vi "niFpgaNotchTemplate.vi"(0 "input data":fxp<+/-,16,16>) -> (4 "output data":fxp<+/-,20,20>)   [LabVIEW 2017]
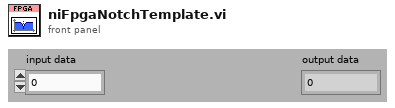
[diagram p1: front panel]
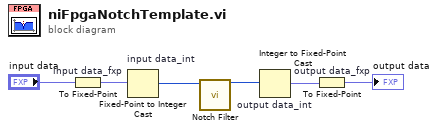
[diagram p0: block diagram]
diagram:
  n1 = To Fixed-Point "input data_fxp"(number="input data") -> (fixed-point=w4:fxp<+/-,16,16>)  [unwired: 1 out]
  n2 = Fixed-Point to Integer Cast "input data_int"(1:w4) -> (0:w1:i16)
  n3 = call "Notch Filter"("input data"=w1) -> ("output data"=w2:i32)  [unwired: 2 in, 12 out]
  n4 = Integer to Fixed-Point Cast "output data_int"(integer=w2) -> (fixed-point=w3:fxp<+/-,32,32>)  [unwired: 1 in]
  n5 = To Fixed-Point "output data_fxp"(number=w3) -> (fixed-point=→"output data":fxp<+/-,20,20>)  [unwired: 1 out]
